vi "create member.vi"() -> ()   [LabVIEW 2023]
uses:
  <resource>/Framework/Providers/LVClassLibrary/NewAccessors/MemberVICreation.lvlib
panel:
  out "error out":errorcluster
  in  "Path":path=path "C:/tmp/fix dll import/generation experiment 1/somelib.lvlib"
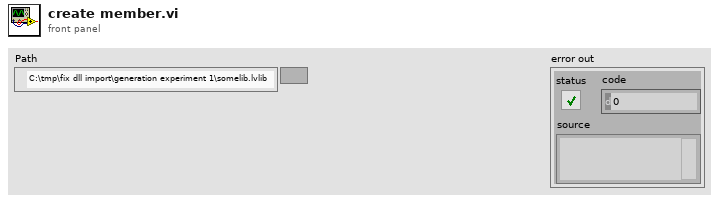
[diagram p1: front panel]
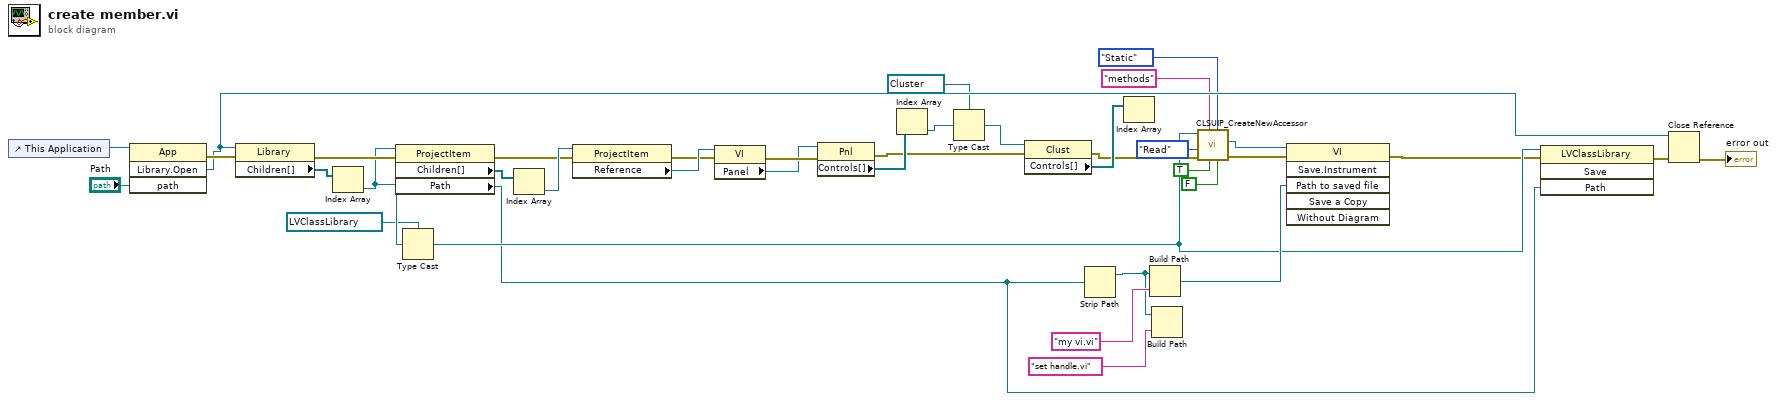
[diagram p0: block diagram]
diagram:
  n1 = control-ref of="This Application"() -> (w38:refnum<vi>)
  n2 = invoke class="App" method="Library.Open"(reference=w38, "path"="Path") -> (error out=w36:errorcluster, "Open Library"=w33:refnum<vi>)  [unwired: 2 in, 2 out]
  n3 = property class="Library"(reference=w33, error in=w36) -> (error out=w32:errorcluster, "Children[]"=w35:refnum<vi>[])  [unwired: 1 out]
  n4 = Index Array(array=w35) -> (element=w22:refnum<vi>)  [unwired: 1 in]
  n5 = property class="ProjectItem"(reference=w22, error in=w32) -> (error out=w20:errorcluster, "Children[]"=w34:refnum<vi>[], "Path"=w5:path)  [unwired: 1 out]
  n6 = Type Cast(type=refnum<vi> refnum ("element"), x=w22) -> (*(type *) &x=w6:refnum<vi>)
  n7 = Index Array(array=w34) -> (element=w31:refnum<vi>)  [unwired: 1 in]
  n8 = property class="ProjectItem"(reference=w31, error in=w20) -> (error out=w19:errorcluster, "Reference"=w30:refnum<vi>)  [unwired: 1 out]
  n9 = property class="VI"(reference=w30, error in=w19) -> (error out=w29:errorcluster, "Panel"=w28:refnum<vi>)  [unwired: 1 out]
  n10 = property class="Pnl"(reference=w28, error in=w29) -> (error out=w18:errorcluster, "Controls[]"=w27:refnum<vi>[])  [unwired: 1 out]
  n11 = Index Array(array=w27) -> (element=w26:refnum<vi>)  [unwired: 1 in]
  n12 = Type Cast(type=refnum<vi> refnum ("element"), x=w26) -> (*(type *) &x=w24:refnum<vi>)
  n13 = property class="Clust"(reference=w24, error in=w18) -> (error out=w17:errorcluster, "Controls[]"=w23:refnum<vi>[])  [unwired: 1 out]
  n14 = Strip Path(path=w5) -> (stripped path=w10:path)  [unwired: 1 out]
  n15 = Index Array(array=w23) -> ()  [unwired: 1 in, 1 out]
  n16 = Build Path(base path=w10, name or relative path="my vi.vi" ("Virtual Folder Name")) -> (appended path=w7:path)
  n17 = Build Path(base path=w10, name or relative path="set handle.vi" ("Virtual Folder Name")) -> ()  [unwired: 1 out]
  n18 = call <resource>:"CLSUIP_CreateNewAccessor.vi"("Make available through Property Nodes"=FALSE, "VI Type"=enum32{"Dynamic", "Static"}."Static", "Include error terminals"=TRUE, "Virtual Folder Name"="methods", "error in (no error)"=w17, "Access UI"=enum16{"Read", "Write", "R/W"}."Read", "LVClassLibrary Ref"=w6) -> ("error out"=w8:errorcluster, "Read VI"=w9:refnum<vi>)  [unwired: 2 in, 1 out]
  n19 = invoke class="VI" method="Save.Instrument"(reference=w9, error in=w8, "Path to saved file"=w7) -> (error out=w1:errorcluster)  [unwired: 3 in, 5 out]
  n20 = invoke class="LVClassLibrary" method="Save"(reference=w6, error in=w1, "Path"=w5) -> (error out=w4:errorcluster)  [unwired: 1 in, 3 out]
  n21 = Close Reference(reference=w33, error in (no error)=w4) -> (error out=→"error out":errorcluster)
